vi "7.1-Make OCU plot.vi"   [LabVIEW 2010]
uses:
  7.0 GUI/7.0 Auto Mode Display.ctl
  7.0-Global.vi
types:
  T1 = typedef "7.0 Auto Mode Display.ctl" = cluster{"Shutdown CMD":bool, "Time":dbl, "Battery":dbl, "Speed (m/s)":dbl, "Heading":dbl, "Latitude":dbl, "Longitude":dbl, "Lattitude of Waypoint":dbl, "Longitude of Waypoint":dbl, "Distance to Waypoint":dbl, "Has Mission Def":bool, "XY Graph":cluster{i32[], "Speed By Path":dbl[]}[]}
  T2 = enum16{"Set Forbrain Act Data", "Read Forebrain Act Data"}
  T3 = typedef "6.1.11- Forbrain and midbrain Act neuron.ctl" = cluster{"4.1- Midbrain Act Data":T4, "6.1.8-Advanced VFH":dbl[]}
  T4 = typedef "4.1-Midbrain Act Data.ctl" = cluster{"Arbitrated Array":sgl[], "Exploded Obstacles":sgl[], "Desired Change in Heading":sgl, "Desired Speed Fraction":sgl}
  T5 = typedef "6.4-How Reporting Typedef.ctl" = cluster{"Drive Speed (m/s)":dbl, "Lidar Inclination (deg) ":dbl, "Steering Angle (deg)":dbl, "Battery Voltage":dbl, "Drive Encoder Cable Check":bool, "Lidar Drive Encoder Cable Check":bool, "Steer Encoder Cable Check":bool, "Lidar Pos Encoder Cable Check":bool, "Mod Buttons & Blinky Cable Check":bool, "Lidar Data Cable Check":bool, "Drive Motor Cable Check":bool, "Vector Nav Cable Check":bool, "Lidar Drive Cable Check":bool, "Steer Drive Cable Check":bool, "Reverse?":bool, "Steering Control Voltage":dbl, "Drive Control Voltage":dbl, "Lidar Control Voltage":dbl}
  T6 = cluster{"Array":sgl[], "Exploded Obstacles":sgl[]}
  T7 = cluster{"Array":sgl[], "6.1.8-Advanced VFH":dbl[]}
  T8 = cluster{"Array":sgl[], "6.1.8-Advanced VFH":dbl[]}[]
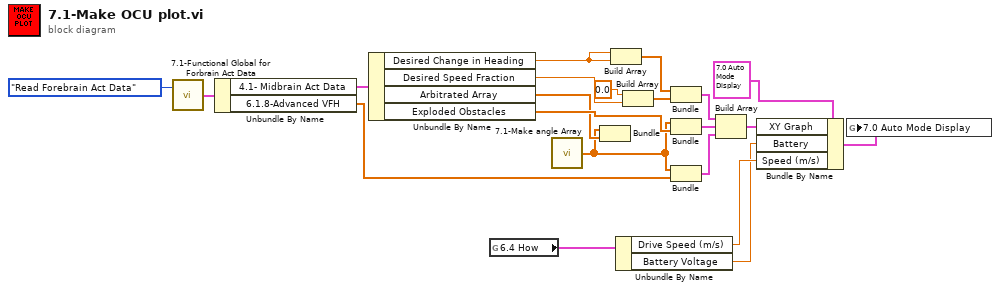
[diagram p0: block diagram]
diagram:
  n1 = call "7.1-Functional Global for Forbrain Act Data.vi"("Command"=T2."Read Forebrain Act Data") -> ("6.1.11-Outputted Forebrain Act Neuron Data"=w20:T3)  [unwired: 1 in]
  n2 = Unbundle By Name(w20) -> ("4.1- Midbrain Act Data"=w14:T4, "6.1.8-Advanced VFH"=w17:dbl[])
  n3 = Unbundle By Name(w14) -> ("Desired Change in Heading"=w8:sgl, "Desired Speed Fraction"=w7:sgl, "Arbitrated Array"=w11:sgl[], "Exploded Obstacles"=w12:sgl[])
  n4 = global read "7.0-Global.vi" "6.4 How"() -> (w3:T5)
  n5 = call "7.1-Make angle Array.vi"() -> ("Array"=w10:sgl[])
  n6 = Bundle("Array"=w10, "Arbitrated Array"=w11) -> ()  [unwired: 1 in, 1 out]
  n7 = Build Array(w8, w8) -> (w9:sgl[])
  n8 = Unbundle By Name(w3) -> ("Drive Speed (m/s)"=w2:dbl, "Battery Voltage"=w1:dbl)
  n9 = Build Array(sgl 0.0 ("element"), w7) -> (w5:sgl[])
  n10 = Bundle(w9, w5) -> (w4:cluster{sgl[], sgl[]})  [unwired: 1 in]
  n11 = Bundle("Array"=w10, "Exploded Obstacles"=w12) -> (w13:T6)  [unwired: 1 in]
  n12 = Bundle("Array"=w10, "6.1.8-Advanced VFH"=w17) -> (w15:T7)  [unwired: 1 in]
  n13 = Build Array(w4, w13, w15) -> (w16:T8)
  n14 = Bundle By Name(cluster=T1 {"Shutdown CMD"=FALSE, "Time"=0.0, "Battery"=0.0, "Speed (m/s)"=0.0, "Heading"=0.0, "Latitude"=0.0, "Longitude"=0.0, "Lattitude of Waypoint"=0.0, "Longitude of Waypoint"=0.0, "Distance to Waypoint"=0.0, "Has Mission Def"=FALSE, "XY Graph"=[]} ("7.0 Auto Mode Display"), "XY Graph"=w16, "Battery"=w1, "Speed (m/s)"=w2) -> (w18:T1)
  n15 = global write "7.0-Global.vi" "7.0 Auto Mode Display"(w18) -> ()
